vi "Read Nested Actors DVR Pool.vi"(11 "Template in":refnum<class "Template.lvclass">) -> (2 "Nested Actors DVR Pool":refnum<queue>[](array[refnum]), 3 "Template out":refnum<class "Template.lvclass">)   [LabVIEW 2020, in "Template.lvlib" / "Template.lvclass"]
uses:
  Template.lvclass
  Template.lvclass/Template.ctl
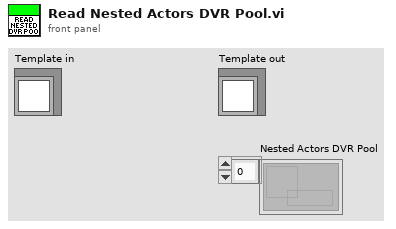
[diagram p1: front panel]
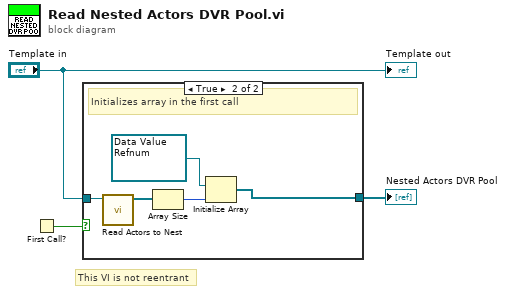
[diagram p0: block diagram]
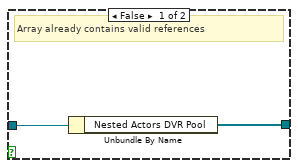
[diagram p2: hidden frame]
diagram:
  # "This VI is not reentrant"
  n1 = First Call?() -> (First Call?: T/F=w2:bool)
  n2 = case shown="True" w2 {
    tunnel: "Template in" -> [w5 w9]
    tunnel: [w4 w6] -> w1
    frame False {
      # "Array already contains valid references"
      n3 = Unbundle By Name(w5) -> ("Nested Actors DVR Pool"=w4:refnum<queue>[])
    }
    frame True {
      # "Initializes array in the first call"
      n4 = call "Read Actors to Nest.vi"("Template in"=w9) -> ("Actors to Nest"=w8:refnum<class "Actor.lvclass">[])  [unwired: 10 in]
      n5 = Array Size(array=w8) -> (size(s)=w10:i32)
      n6 = Initialize Array(refnum<queue> refnum ("DVR Pool"), w10) -> (w6:refnum<queue>[])
    }
  }
  "Nested Actors DVR Pool" <- w1
  "Template out" <- "Template in"
